vi "WPI_CameraOpen Internal.vi"(8 "error in (no error)":errorcluster, 11 "Camera Address":string="192.168.0.90") -> (0 "error out":errorcluster, 3 "CameraDevRef":T1)   [LabVIEW 2017]
doc: "This software is licensed. Open the labview\\readme\\WPI Robotics Library Open Source License.txt file for more information."
uses:
  <vilib>/Rock Robotics/WPI/Camera/WPI_CameraDevRef.ctl
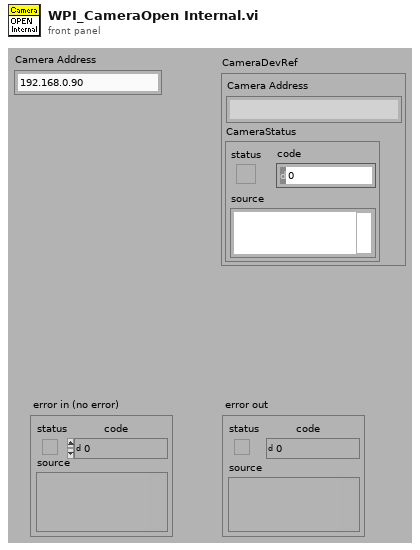
[diagram p1: front panel]
types:
  T1 = typedef "WPI_CameraDevRef.ctl" = cluster{"Camera Address":string, "CameraStatus":errorcluster}
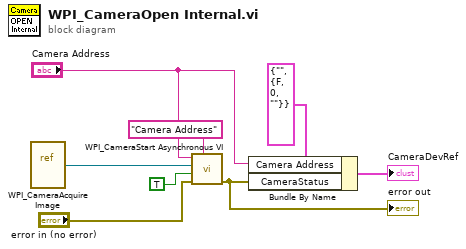
[diagram p0: block diagram]
diagram:
  n1 = vi-ref <vilib>:"WPI_CameraAcquire Image.vi"() -> (w8:refnum<vi>)
  n2 = call <vilib>:"WPI_CameraStart Asynchronous VI.vi"("Control Name"="Camera Address", "error in (no error)"="error in (no error)", "Auto Dispose Reference"=TRUE, "VI Refnum"=w8, "Value"="Camera Address") -> ("error out"=w2:errorcluster)  [unwired: 6 out]
  "error out" <- w2
  n3 = Bundle By Name(cluster=T1 {"Camera Address"="", "CameraStatus"={"status"=FALSE, "code"=0, "source"=""}} ("CameraDevRef"), "Camera Address"="Camera Address", "CameraStatus"=w2) -> (→"CameraDevRef":T1)
